vi "Counter.vi"(10 "Input Valid":bool=TRUE, 11 "Counter End  Value":u32) -> (2 "Counter Value":u32, 3 "End Reached":bool)   [LabVIEW 2013]
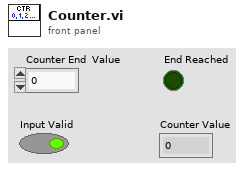
[diagram p1: front panel]
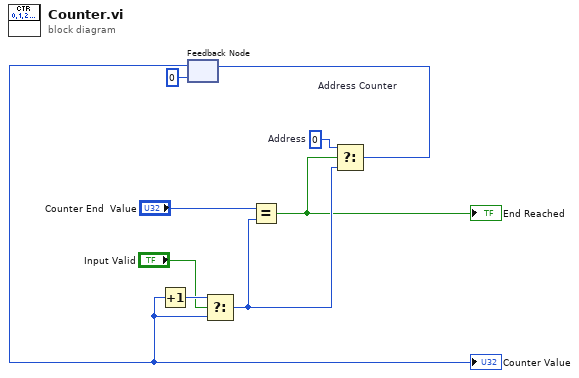
[diagram p0: block diagram]
diagram:
  w9 = u32 0  # Address
  n1 = feedback #1 "Address Counter"(u32 0 ("Address")) -> (w2:u32)
  "Counter Value" <- w2
  n2 = Increment(x=w2) -> (x+1=w6:u32)
  n3 = Select(t=w6, s="Input Valid", f=w2) -> (s? t:f=w5:u32)
  n4 = Equal?(x="Counter End  Value", y=w5) -> (x = y?=w1:bool)
  "End Reached" <- w1
  n5 = Select(t=w9, s=w1, f=w5) -> (s? t:f=w8:u32)
  n6 = feedback-in #1(w8) -> ()
